vi "QTrkSpeedTest.vi"(6 "LUT (in)":dbl[][](graph)=array200x64[12800 elements], 8 "ZLUT planes":i32=50, 9 "2D Localization Type":T1=enum."Quadrant Interpolation", 10 "Z Localization?":bool=TRUE, 11 "QTrk Settings":T3={"Image width"=80, "Image height"=80, "Number of threads (CPU based)"=-1, "CUDA Device"=-2, "COM Background correction factor"=0.0, "ZLUT MinRadius"=2.0, "ZLUT Radial sample density"=5.0, "ZLUT Angular sample density"=2.0, "ZLUT ROI Coverage"=0.7, "QI Iterations"=3, "QI MinRadius"=4.0, "QI Radial sample density"=2.0, "QI Angular sample density"=3.0, "QI ROI Coverage"=1.0, "QI Angular Step \nIteration Factor"=0.8, "XCOR Profile Length"=1, "XCOR Profile Width"=128, "XCOR Iterations"=32, "Gaussian 2D Fit Iterations"=2, "Gaussian 2D Sigma (pixels)"=3.0, "Downsample"=0} {"QI Angular Step \nIteration Factor" format="%_3f"; "ZLUT ROI Coverage" format="%#_3g"; "QI ROI Coverage" format="%#_3g"; "QI MinRadius" format="%#_3g"; "QI Angular sample density" format="%#_3g"; "QI Radial sample density" format="%#_3g"; "QI Iterations" format="%_3f"; "ZLUT Angular sample density" format="%#_3g"; "ZLUT Radial sample density" format="%#_3g"; "XCOR Profile Length" format="%_3f"}) -> (1 "ZLUT":sgl[][](graph), 3 "Images/s":dbl)   [LabVIEW 2011]
uses:
  QTrkZCommandType.ctl
  QTrkSettings.ctl
  QTrkLocalizationType.ctl
panel:
  out "debug image":sgl[][](graph)
  in  "Debug: Save LUT images?":bool
  out "Derived settings":T2
  out "Queue length":i32
  out "Queue capacity used %":dbl format="%#.2f"
  out "report":string
  out "Test Image":u8[][](graph)
  out "Images processed:":i32
  out "Image count:":i32=4000
  # "Running speed test...."
  # "-2: Use all devices\n-1: Use best device"
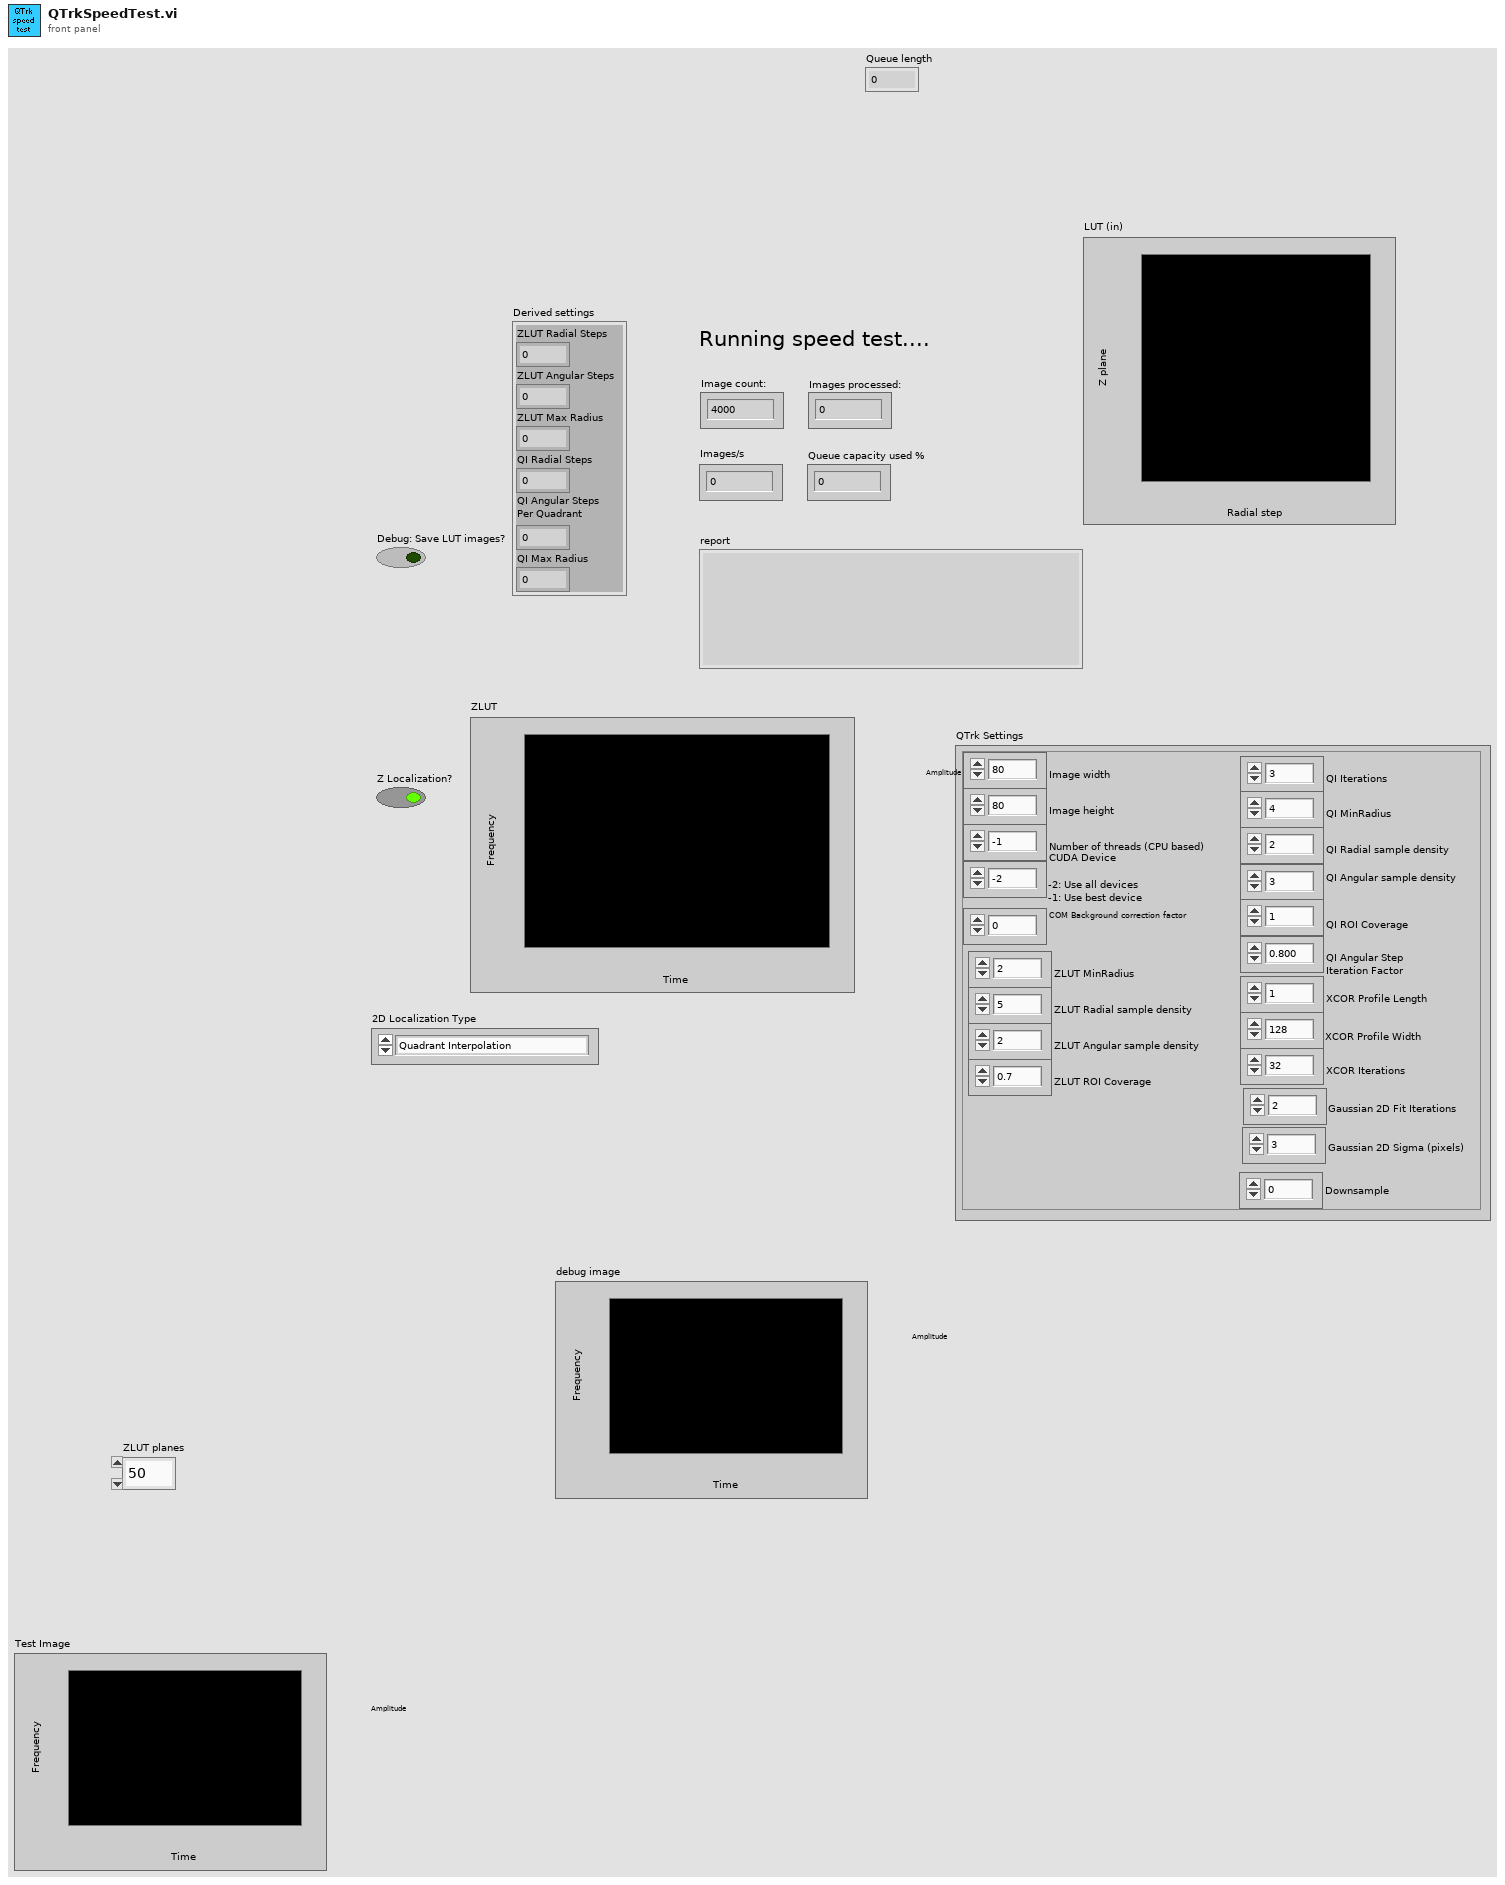
[diagram p1: front panel]
types:
  T1 = typedef "QTrkLocalizationType.ctl" = enum16{"Center-of-Mass", "1D Cross-Correlation", "Quadrant Interpolation", "Gaussian 2D MLE", "QI + ZLUTAlign", "ZLUTAlign", "QI + FourierLUT"}
  T2 = cluster{"ZLUT Radial Steps":i32, "ZLUT Angular Steps":i32, "ZLUT Max Radius":sgl, "QI Radial Steps":i32, "QI Angular Steps\nPer Quadrant":i32, "QI Max Radius":sgl}
  T3 = typedef "QTrkSettings.ctl" = cluster{"Image width":i32, "Image height":i32, "Number of threads (CPU based)":i32, "CUDA Device":i32, "COM Background correction factor":sgl, "ZLUT MinRadius":sgl, "ZLUT Radial sample density":sgl, "ZLUT Angular sample density":sgl, "ZLUT ROI Coverage":sgl, "QI Iterations":i32, "QI MinRadius":sgl, "QI Radial sample density":sgl, "QI Angular sample density":sgl, "QI ROI Coverage":sgl, "QI Angular Step \nIteration Factor":sgl, "XCOR Profile Length":i32, "XCOR Profile Width":i32, "XCOR Iterations":i32, "Gaussian 2D Fit Iterations":i32, "Gaussian 2D Sigma (pixels)":sgl, "Downsample":i32}
  T4 = typedef "QTrkZCommandType.ctl" = enum16{"Nothing", "ComputeZ"}
  T5 = typedef "QTrkInstance.ctl" = cluster{"QTrk Pointer":u64}
  T6 = typedef "QTrkComputedSettings.ctl" = cluster{"QTrk Settings":T3, "Derived settings":cluster{"ZLUT Radial Steps":i32, "ZLUT Angular Steps":i32, "ZLUT Max Radius":sgl, "QI Radial Steps":i32, "QI Angular Steps\nPer Quadrant":i32, "QI Max Radius":sgl}}
  T7 = cluster{"ZLUT MinRadius":sgl, "ZLUT Max Radius":sgl}
  T8 = typedef "IMAQ Image.ctl" = refnum<image>
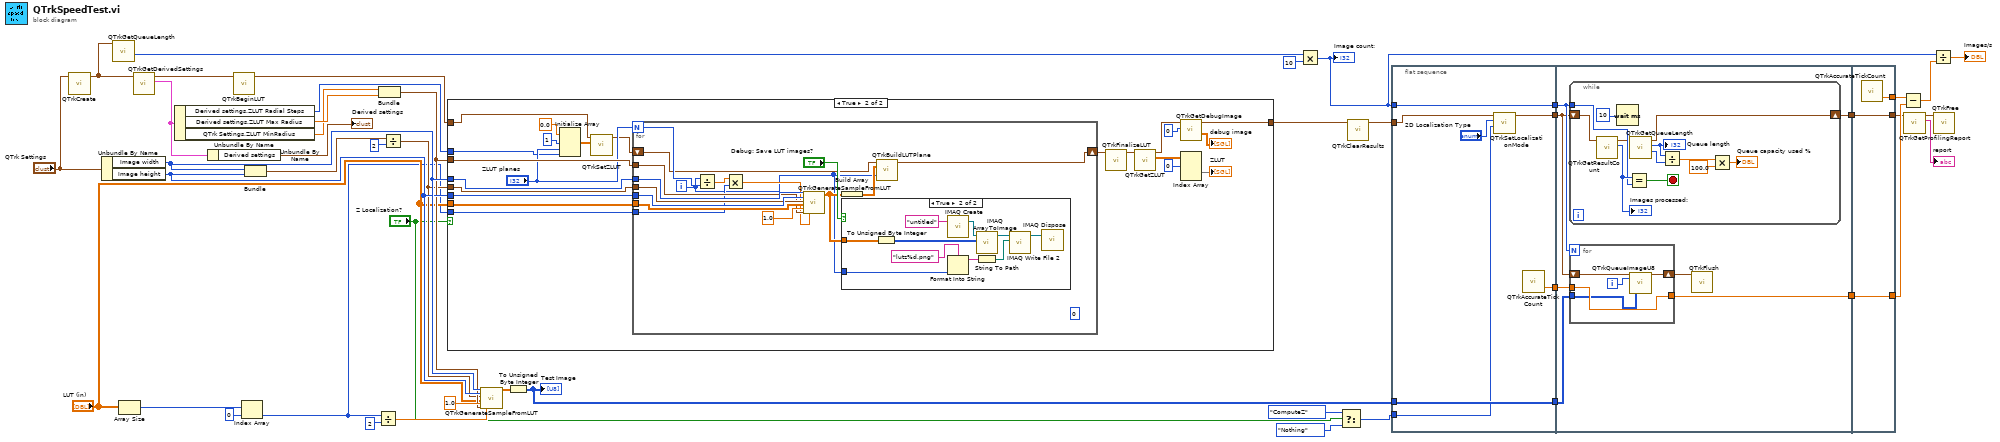
[diagram p0: block diagram]
diagram:
  n1 = call "QTrkCreate.vi"("QTrk Settings"="QTrk Settings") -> ("QTrk Instance"=w17:T5)  [unwired: 4 in, 2 out]
  n2 = Unbundle By Name("QTrk Settings") -> ("Image width"=w37:i32, "Image height"=w36:i32)
  n3 = call "QTrkGetQueueLength.vi"("QTrk Instance"=w17) -> ("maxQueueLen"=w16:i32)  [unwired: 7 in, 3 out]
  n4 = Array Size(array="LUT (in)") -> (size(s)=w31:i32[])
  n5 = call "QTrkGetDerivedSettings.vi"("QTrk Instance"=w17) -> ("Derived settings"=w11:T6, "QTrk Instance (out)"=w2:T5)  [unwired: 5 in, 4 out]
  n6 = Unbundle By Name(w11) -> ("Derived settings.ZLUT Radial Steps"=w18:i32, "Derived settings.ZLUT Max Radius"=w42:sgl, "QTrk Settings.ZLUT MinRadius"=w41:sgl)
  n7 = Unbundle By Name(w11) -> ("Derived settings"=→"Derived settings":T2)
  n8 = call "QTrkBeginLUT.vi"("QTrk Instance"=w2) -> ("QTrk Instance"=w1:T5)  [unwired: 5 in, 1 out]
  n9 = Index Array(array=w31, index=0) -> (element=w27:i32)
  n10 = Bundle("Image width"=w37, "Image height"=w36) -> (w44:cluster{"Image width":i32, "Image height":i32})  [unwired: 1 in]
  n11 = Divide(x=w27, y=2) -> (x/y=w28:dbl)
  n12 = Bundle("ZLUT MinRadius"=w41, "ZLUT Max Radius"=w42) -> (w34:T7)  [unwired: 1 in]
  n13 = Divide(x=w44, y=2 ("Image height")) -> (x/y=w33:cluster{"Image width":dbl, "Image height":dbl})
  n14 = case shown="True" "Z Localization?" {
    tunnel: w37 -> [_ w66]
    tunnel: w36 -> [_ w65]
    tunnel: w34 -> [_ w64]
    tunnel: w33 -> [_ w63]
    tunnel: "LUT (in)" -> [_ w62]
    tunnel: w27 -> [_ w61]
    tunnel: w1 -> [w47 w60]
    tunnel: w18 -> [_ w55]
    tunnel: [w47 w51] -> w7
    frame False {
    }
    frame True {
      n15 = Initialize Array(0.0 ("element"), 1 ("dimension size"), "ZLUT planes", w55) -> (w59:dbl[][][])
      n16 = call "QTrkSetZLUT.vi"("ZLUT"=w59, "QTrk Instance"=w60) -> ("QTrk Instance"=w54:T5)  [unwired: 8 in, 1 out]
      n17 = for {
        N: "ZLUT planes" -> [w79]
        shift-right: [w70] -> w49
        shift-left: w54 -> [w71]
        tunnel: w66 -> [w85]
        tunnel: w65 -> [w84]
        tunnel: w63 -> [w83]
        tunnel: w62 -> [w82]
        tunnel: w64 -> [w80]
        tunnel: w61 -> [w77]
        i -> [w72]
        (unwired) 0 ("zlutIndex")
        n18 = Divide(x=w72, y=w79) -> (x/y=w78:dbl)
        n19 = Multiply(x=w78, y=w77) -> (x*y=w76:dbl)
        n20 = call "QTrkGenerateSampleFromLUT.vi"("Width"=w85, "Height"=w84, "position"=w83, "LUT"=w82, "magnification"=sgl 1.0, "LUT radii"=w80, "z"=w76) -> ("image"=w74:sgl[][])  [unwired: 12 in]
        n21 = Build Array(w74) -> (w73:sgl[][][])
        n22 = case shown="True" "Debug: Save LUT images?" {
          tunnel: w74 -> [_ w94]
          tunnel: w72 -> [_ w89]
          frame False {
          }
          frame True {
            n23 = To Unsigned Byte Integer(number=w94) -> (unsigned 8bit integer=w93:u8[][])
            n24 = call "IMAQ Create"("Image Name"="untitled") -> ("New Image"=w95:T8)  [unwired: 4 in, 1 out]
            n25 = Format Into String(format string="lutz%d.png", w89) -> (resulting string=w88:string)  [unwired: 2 in, 1 out]
            n26 = String To Path(string=w88) -> (path=w87:path)
            n27 = call "IMAQ ArrayToImage"("Image Pixels (U8)"=w93, "Image"=w95) -> ("Image Out"=w92:T8)  [unwired: 8 in, 1 out]
            n28 = call-poly "IMAQ Write File 2"("File Path"=w87, "Image"=w92) -> ("Image Out (duplicate)"=w91:T8)  [unwired: 8 in, 1 out]
            n29 = call "IMAQ Dispose"("Image"=w91) -> ()  [unwired: 5 in, 1 out]
          }
        }
        n30 = call "QTrkBuildLUTPlane.vi"("QTrk Instance"=w71, "Bead images"=w73, "plane"=w72) -> ("QTrk Instance"=w70:T5)  [unwired: 11 in, 1 out]
      }
      n31 = call "QTrkFinalizeLUT.vi"("QTrk Instance"=w49) -> ("QTrk Instance"=w48:T5)  [unwired: 5 in, 1 out]
      n32 = call "QTrkGetZLUT.vi"("QTrk Instance (in)"=w48) -> ("zlut"=w69:sgl[][][], "QTrk Instance"=w52:T5)  [unwired: 8 in, 1 out]
      n33 = call "QTrkGetDebugImage.vi"("id"=0, "QTrk Instance"=w52) -> ("data"=→"debug image":sgl[][], "QTrk Instance (out)"=w51:T5)  [unwired: 7 in, 1 out]
      n34 = Index Array(array=w69, index (dim 0)=0 ("index (page)")) -> (element=→"ZLUT":sgl[][])  [unwired: 2 in]
    }
  }
  n35 = call "QTrkGenerateSampleFromLUT.vi"("Width"=w37, "Height"=w36, "position"=w33, "LUT"="LUT (in)", "magnification"=sgl 1.0, "LUT radii"=w34, "z"=w28) -> ("image"=w19:sgl[][])  [unwired: 12 in]
  n36 = To Unsigned Byte Integer(number=w19) -> (unsigned 8bit integer=w9:u8[][])
  "Test Image" <- w9
  n37 = Multiply(x=w16, y=10) -> (x*y=w14:i32)
  "Image count:" <- w14
  n38 = Select(t=QTrkZCommandType."ComputeZ" ("Z Command"), s="Z Localization?", f=QTrkZCommandType."Nothing" ("Z Command")) -> (s? t:f=w3:T4)
  n39 = call "QTrkClearResults.vi"("QTrk Instance (in)"=w7) -> ("QTrk Instance (out)"=w46:T5)  [unwired: 9 in, 1 out]
  n40 = flat-sequence {
    tunnel: w9 -> [w101]
    tunnel: w14 -> [w102]
    tunnel: w46 -> [w99]
    tunnel: [w98] -> w26
    tunnel: [w100] -> w25
    tunnel: [w102] -> w24
    tunnel: [w101] -> w23
    tunnel: w3 -> [w97]
    tunnel: w26 -> [w104]
    tunnel: w25 -> [w108]
    tunnel: w24 -> [w105]
    tunnel: w23 -> [w103]
    tunnel: [w109] -> w22
    tunnel: [w106] -> w21
    tunnel: [w128] -> w13
    tunnel: [w129] -> w40
    tunnel: w22 -> [w129]
    tunnel: w21 -> [w128]
    tunnel: [w127] -> w20
    frame #0 {
      n41 = call "QTrkSetLocalizationMode.vi"("Z Command"=w97, "2D Localization Type"="2D Localization Type", "QTrk Instance"=w99) -> ("QTrk Instance"=w98:T5)  [unwired: 8 in]
      n42 = call "QTrkAccurateTickCount.vi"() -> ("seconds"=w100:dbl)  [unwired: 2 in, 1 out]
    }
    frame #1 {
      n43 = while {
        shift-right: [w115] -> w106
        shift-left: w104 -> [w121]
        tunnel: w105 -> [w119]
        stop <- w118 stop-if-true
        n44 = call "QTrkGetResultCount.vi"("QTrk Instance"=w121) -> ("result count"=w120:i32, "QTrk Instance"=w116:T5)  [unwired: 4 in, 1 out]
        "Images processed:" <- w120
        n45 = Wait (ms)(milliseconds to wait=u32 10) -> ()  [unwired: 1 out]
        n46 = Equal?(x=w120, y=w119) -> (x = y?=w118:bool)
        n47 = call "QTrkGetQueueLength.vi"("QTrk Instance"=w116) -> ("maxQueueLen"=w113:i32, "queue size"=w114:i32, "QTrk Instance"=w115:T5)  [unwired: 7 in, 1 out]
        "Queue length" <- w114
        n48 = Divide(x=w114, y=w113) -> (x/y=w111:dbl)
        n49 = Multiply(x=w111, y=100.0) -> (x*y=→"Queue capacity used %":dbl)
      }
      n50 = for {
        N: w105 -> [_]
        shift-right: [w122] -> w107
        shift-left: w104 -> [w126]
        tunnel: w108 -> [w125]
        tunnel: [w125] -> w109
        tunnel: w103 -> [w124]
        i -> [w123]
        n51 = call "QTrkQueueImageU8.vi"("QTrk Instance"=w126, "frame"=w123, "image"=w124) -> ("QTrk Instance"=w122:T5)  [unwired: 15 in, 1 out]
      }
      n52 = call "QTrkFlush.vi"("QTrk Instance"=w107) -> ()  [unwired: 9 in, 2 out]
    }
    frame #2 {
      n53 = call "QTrkAccurateTickCount.vi"() -> ("seconds"=w127:dbl)  [unwired: 2 in, 1 out]
    }
  }
  n54 = Subtract(x=w20, y=w40) -> (x-y=w39:dbl)
  n55 = call "QTrkGetProfilingReport.vi"("QTrk Instance"=w13) -> ("report"=→"report":string, "QTrk Instance (out)"=w8:T5)  [unwired: 9 in]
  n56 = Divide(x=w14, y=w39) -> (x/y=→"Images/s":dbl)
  n57 = call "QTrkFree.vi"("QTrk Instance"=w8) -> ()  [unwired: 6 in, 1 out]
